vi "DAQmx.Recovery Error Handler.vi"(8 "error in (no error)":errorcluster, 11 "DAQmx in":refnum<class "DAQmx.lvclass">) -> (0 "error out":errorcluster, 2 "retry?":bool, 3 "DAQmxout":refnum<class "DAQmx.lvclass">)   [LabVIEW 2019, in "DAQmx.lvclass"]
uses:
  DAQmx.lvclass
  DAQmx.lvclass/DAQmx.ctl
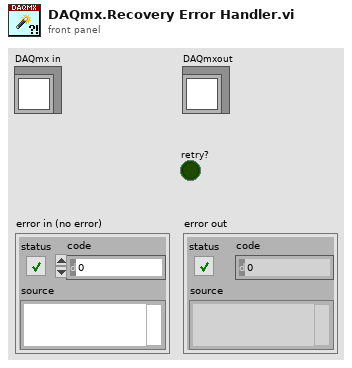
[diagram p1: front panel]
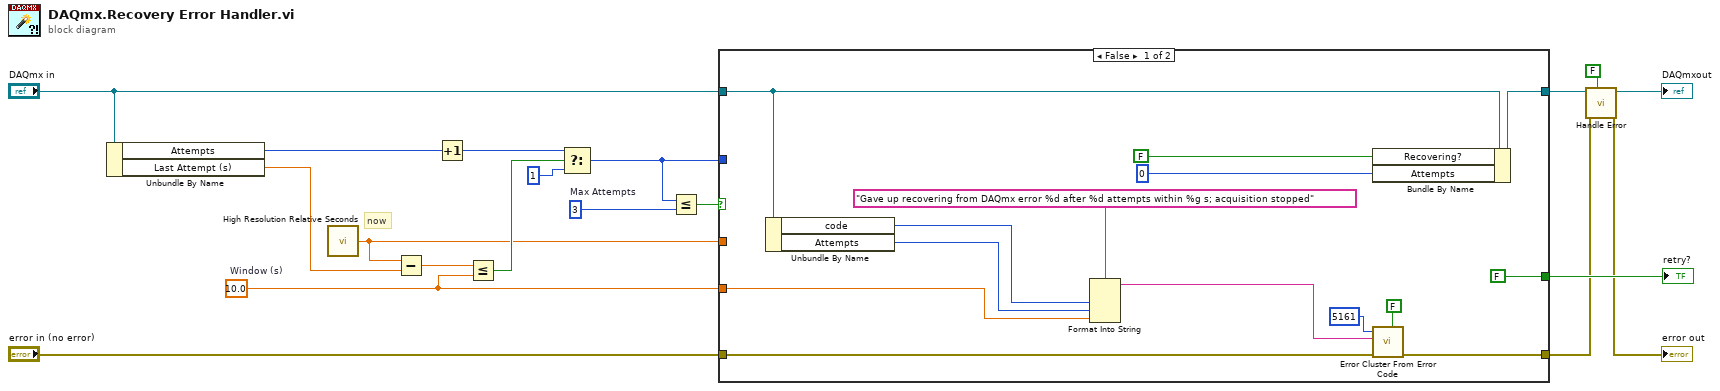
[diagram p0: block diagram]
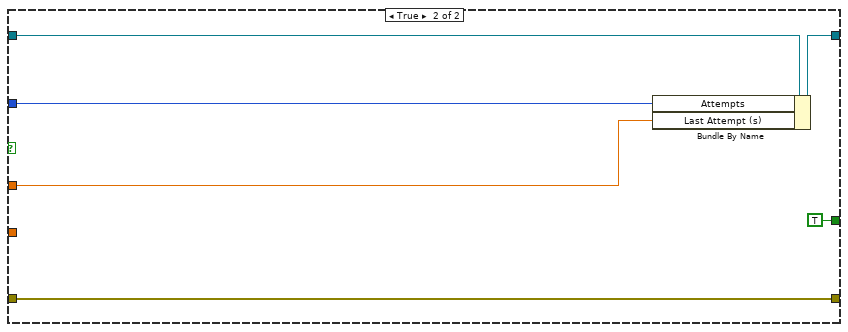
[diagram p2: hidden frame]
diagram:
  w3 = 10.0  # Window (s)
  w19 = 3  # Max Attempts
  # "now"
  n1 = Unbundle By Name("DAQmx in") -> ("Attempts"=w8:i32, "Last Attempt (s)"=w9:dbl)
  n2 = call <vilib>:"High Resolution Relative Seconds.vi"() -> ("relative seconds"=w1:dbl)
  n3 = Subtract(x=w1, y=w9) -> (x-y=w7:dbl)
  n4 = Increment(x=w8) -> (x+1=w5:i32)
  n5 = Less Or Equal?(x=w7, y=w3) -> (x <= y?=w6:bool)
  n6 = Select(t=w5, s=w6, f=1) -> (s? t:f=w2:i32)
  n7 = Less Or Equal?(x=w2, y=w19) -> (x <= y?=w17:bool)
  n8 = case shown="False" w17 {
    tunnel: [FALSE TRUE] -> w18
    tunnel: w3 -> [w21 _]
    tunnel: "error in (no error)" -> [w28 w38]
    tunnel: [w27 w38] -> w13
    tunnel: "DAQmx in" -> [w25 w36]
    tunnel: [w26 w39] -> w15
    tunnel: w2 -> [_ w35]
    tunnel: w1 -> [_ w34]
    frame False {
      n9 = Unbundle By Name(w25) -> ("code"=w23:i32, "Attempts"=w24:i32)
      n10 = Format Into String(format string="Gave up recovering from DAQmx error %d after %d attempts within %g s; acquisition stopped", w23, w24, w21) -> (resulting string=w29:string)  [unwired: 2 in, 1 out]
      n11 = Bundle By Name(cluster=w25, "Recovering?"=FALSE ("Recovery.Recovering?"), "Attempts"=0 ("Recovery.Attempts")) -> (w26:refnum<class "DAQmx.lvclass">)
      n12 = call <vilib>:"Error Cluster From Error Code.vi"("is warning? (False)"=FALSE, "error in (no error)"=w28, "error message (\"\")"=w29, "error code (0)"=5161 ("code")) -> ("error out"=w27:errorcluster)  [unwired: 5 in]
    }
    frame True {
      n13 = Bundle By Name(cluster=w36, "Attempts"=w35, "Last Attempt (s)"=w34) -> (w39:refnum<class "DAQmx.lvclass">)
    }
  }
  "retry?" <- w18
  n14 = call-dynamic "Handle Error.vi"("Stop on Unhandled Error (T)"=FALSE, "error in"=w13, "DAQmx"=w15) -> ("handling error"=→"error out":errorcluster, "DAQmx out"=→"DAQmxout":refnum<class "DAQmx.lvclass">)  [unwired: 6 in, 1 out]
